vi "PumpDispense_num.vi"(8 "Error In":errorcluster, 9 "Flowrate(ul/min)":dbl, 10 "Pump Address":dbl, 11 "Pump COMM Port":refnum<visa-resource-name>) -> (0 "Error Out":errorcluster, 3 "Pump COMM Port Out":refnum<visa-resource-name>)   [LabVIEW 2014]
panel:
  # "Dispense Micro Lynx Milligat Pumps"
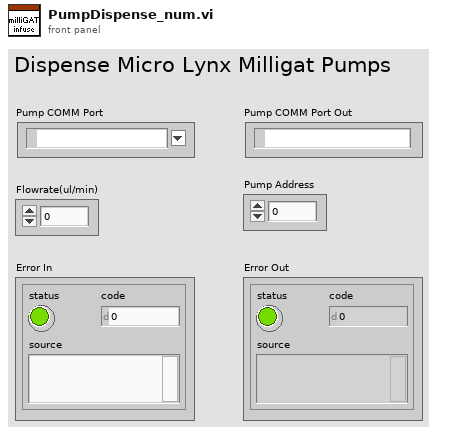
[diagram p1: front panel]
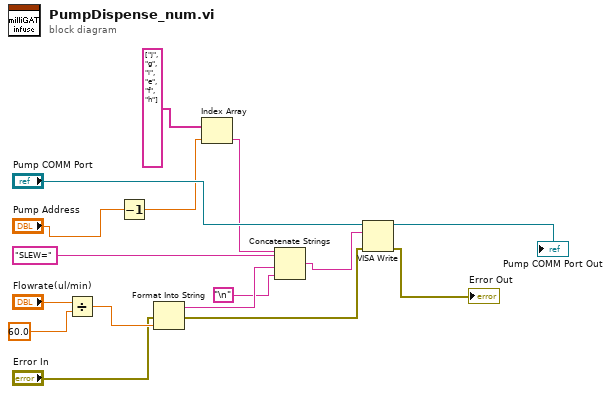
[diagram p0: block diagram]
diagram:
  n1 = Divide(x="Flowrate(ul/min)", y=60.0) -> (x/y=w13:dbl)
  n2 = Decrement(x="Pump Address") -> (x-1=w2:dbl)
  n3 = Format Into String(error in="Error In", w13) -> (resulting string=w7:string, error out=w11:errorcluster)  [unwired: 2 in]
  n4 = Index Array(array=string[] ["j", "g", "i", "e", "f", "h"], index=w2) -> (element=w1:string)
  n5 = Concatenate Strings(w1, "SLEW=", w7, "\n") -> (w9:string)
  n6 = VISA Write(VISA resource name="Pump COMM Port", write buffer=w9, error in (no error)=w11) -> (VISA resource name out=→"Pump COMM Port Out":refnum<visa-resource-name>, error out=→"Error Out":errorcluster)  [unwired: 1 out]
